vi "From String Test.vi"() -> (0 "error out":errorcluster, 2 "View Name Matches":bool)   [LabVIEW 2014, in "Missing Plugin tests.lvlib"]
doc: "Test Missing \"Missing Plugin configuration.from string\" function. VI should return with no error for any flattened module."
uses:
  Missing Plugin tests.lvlib
  module/configuration/Missing Plugin configuration.lvclass
  <vilib>/NI/Configuration Framework/serializable configuration/NISE_CEF_serializable configuration.lvclass
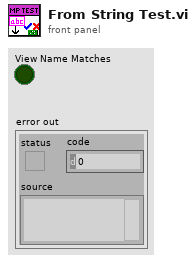
[diagram p1: front panel]
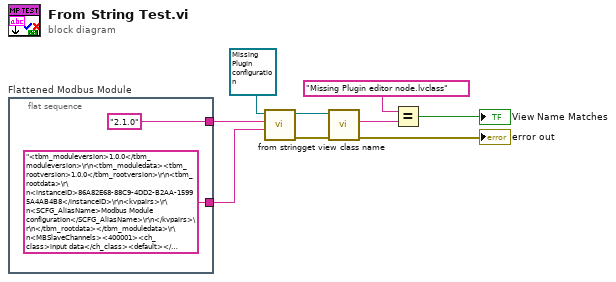
[diagram p0: block diagram]
diagram:
  n1 = flat-sequence "Flattened Modbus Module" {
    tunnel: ["2.1.0" ("version")] -> w9
    tunnel: ["<tbm_moduleversion>1.0.0</tbm_moduleversion>\r\n<tbm_moduledata><tbm_rootversion>1.0.0</tbm_rootversion>\r\n<tbm_rootdata>\r\n<instanceID>86A82E68-88C9-4DD2-B2AA-15995A4AB4B8</instanceID>\r\n<kvpairs>\r\n<SCFG_AliasName>Modbus Module configuration</SCFG_AliasName>\r\n</kvpairs>\r\n</tbm_rootdata></tbm_moduledata>\r\n<MBSlaveChannels><400001><ch_class>input data</ch_class><default></default><meta></meta><ch_type>U16</ch_type><ch_version>1.0.0</ch_version><mbc_mbtype>holding registers</mbc_mbtype><mbc_startaddr>0</mbc_startaddr><mbc_subindex>0</mbc_subindex></400001>\r\n<400002><ch_class>output data</ch_class><default></default><meta></meta><ch_type>U16</ch_type><ch_version>1.0.0</ch_version><mbc_mbtype>holding registers</mbc_mbtype><mbc_startaddr>1</mbc_startaddr><mbc_subindex>0</mbc_subindex></400002>\r\n<000003><ch_class>input data</ch_class><default></default><meta></meta><ch_type>Boolean</ch_type><ch_version>1.0.0</ch_version><mbc_mbtype>coils</mbc_mbtype><mbc_startaddr>2</mbc_startaddr><mbc_subindex>0</mbc_subindex></000003>\r\n<000004><ch_class>output data</ch_class><default></default><meta></meta><ch_type>Boolean</ch_type><ch_version>1.0.0</ch_version><mbc_mbtype>coils</mbc_mbtype><mbc_startaddr>3</mbc_startaddr><mbc_subindex>0</mbc_subindex></000004>\r\n</MBSlaveChannels>\r\n<MBSlavePort>502</MBSlavePort>\r\n<MBFlowCtl>0</MBFlowCtl>\r\n<MBSerADU>RTU</MBSerADU>\r\n<MBParity>2</MBParity>\r\n<MBUnitID>1</MBUnitID>\r\n<MBBaudRate>9600</MBBaudRate>\r\n<MBVisaResource></MBVisaResource>\r\n<MBClass>TCP master</MBClass>\r\n<MBTCPAddr></MBTCPAddr>\r\n<MBSERForceWireMode>FALSE</MBSERForceWireMode>\r\n<MBSERWireMode>0</MBSERWireMode><MBFirstWordLow>FALSE</MBFirstWordLow><MBFirstDWordLow>FALSE</MBFirstDWordLow>" ("version")] -> w8
    frame #0 {
    }
  }
  n2 = call-dynamic "from string.vi"("data"=w8, "version"=w9, "Missing Plugin configuration in"=refnum<class "Missing Plugin configuration.lvclass"> refnum) -> ("error out"=w5:errorcluster, "Missing Plugin configuration out"=w6:refnum<class "Missing Plugin configuration.lvclass">)  [unwired: 7 in]
  n3 = call <vilib>:"get view class name.vi"("error in"=w5, "configuration in"=w6) -> ("error out"=→"error out":errorcluster, "view class"=w4:string)  [unwired: 7 in, 1 out]
  n4 = Equal?(x="Missing Plugin editor node.lvclass", y=w4) -> (x = y?=→"View Name Matches":bool)
